vi "Close.vi"(8 "error in (no error)":errorcluster, 11 "Carya Config (Buffer) in":refnum<class "CConfig By Ref Buffer.lvclass">) -> (0 "error out":errorcluster)   [LabVIEW 2013, in "CConfig By Ref Buffer.lvclass"]
doc: "Copyright 2018, Carya Automatisering, Wiebe Walstra."
uses:
  CConfig By Ref Buffer.lvclass
  Buffer Functions.ctl
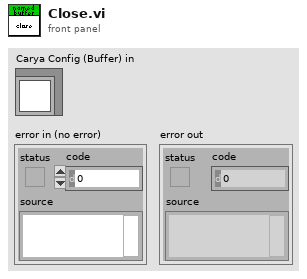
[diagram p1: front panel]
types:
  T1 = typedef "CConfig By Ref Buffer.lvclass/Buffer Functions.ctl" = enum16{"register", "get and lock", "set and unlock", "unlock", "unregister", "check"}
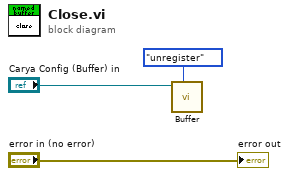
[diagram p0: block diagram]
diagram:
  n1 = call "Buffer.vi"("Functions"=Buffer_Functions."unregister", "Carya Config (Buffer) in"="Carya Config (Buffer) in") -> ()  [unwired: 5 in, 5 out]
  "error out" <- "error in (no error)"
